vi "Constructor by Info Cluster Text.vi"(8 "error in (no error)":errorcluster, 9 "Text Field Info":T1, 10 "Database (use member data)":refnum<class "Database.lvclass">, 11 "Field in":refnum<class "Field.lvclass">) -> (0 "error out":errorcluster, 3 "Field out":refnum<class "Field.lvclass">)   [LabVIEW 2020, in "Old Field.lvlib" / "Field.lvclass"]
uses:
  Field.lvclass
  Database Libraries/Database/Database Class/Database.lvclass
  Text Field Info.ctl
  Basic Fields/Text field Class/Text field.lvclass
  C:/Users/User/Desktop/Raman Program/Database OOP/source/Database OOP/Field/Field Class/Field.lvclass
  Field.lvclass/Field.ctl
  Old Field.lvlib
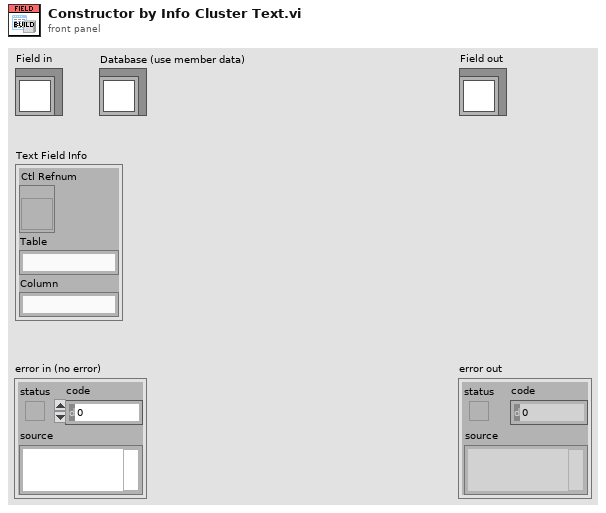
[diagram p1: front panel]
types:
  T1 = typedef "Old Field.lvlib/Text Field Info.ctl" = cluster{"Ctl Refnum":refnum<vi>, "Table":string, "Column":string}
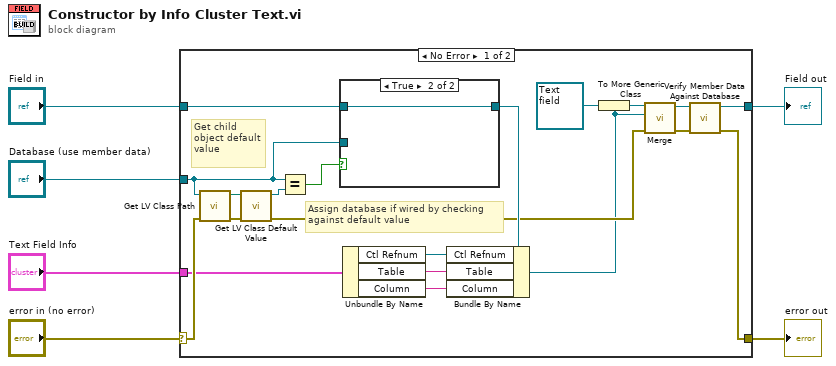
[diagram p0: block diagram]
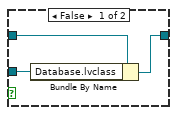
[diagram p2: hidden frame]
diagram:
  n1 = case shown="No Error" "error in (no error)" {
    selector: "error in (no error)" -> [w20 w32]
    tunnel: [w8 w32] -> w5
    tunnel: [w7 w31] -> w3
    tunnel: "Field in" -> [w21 w31]
    tunnel: "Database (use member data)" -> [w22 _]
    tunnel: "Text Field Info" -> [w17 _]
    frame No Error {
      # "Get child object default value"
      # "Assign database if wired by checking\nagainst default value"
      n2 = call <vilib>:"Get LV Class Path.vi"("error in (no error)"=w20, "object"=w22) -> ("error out"=w25:errorcluster, "class path"=w26:path)  [unwired: 8 in]
      n3 = call <vilib>:"Get LV Class Default Value.vi"("error in (no error)"=w25, "class path"=w26) -> ("error out"=w18:errorcluster, "object"=w24:refnum<class>)  [unwired: 8 in]
      n4 = Equal?(x=w22, y=w24) -> (x = y?=w23:bool)
      n5 = case shown="True" w23 {
        tunnel: w22 -> [w28 _]
        tunnel: w21 -> [w29 w30]
        tunnel: [w27 w30] -> w19
        frame False {
          n6 = Bundle By Name(cluster=w29, "Database.lvclass"=w28) -> (w27:refnum<class "Field.lvclass">)
        }
        frame True {
        }
      }
      n7 = Unbundle By Name(w17) -> ("Ctl Refnum"=w16:refnum<vi>, "Table"=w15:string, "Column"=w14:string)
      n8 = Bundle By Name(cluster=w19, "Ctl Refnum"=w16, "Table"=w15, "Column"=w14) -> (w12:refnum<class "Field.lvclass">)
      n9 = To More Generic Class(target class=w12, reference=refnum<class "Text field.lvclass"> refnum ("Text field.lvclass")) -> (generic class reference=w13:refnum<class "Field.lvclass">)
      n10 = call-dynamic "Merge.vi"("error in (no error)"=w18, "Field To Merge"=w12, "Field In"=w13) -> ("error out"=w9:errorcluster, "Merged Field out"=w10:refnum<class "Field.lvclass">)  [unwired: 7 in]
      n11 = call-dynamic "Verify Member Data Against Database.vi"("error in (no error)"=w9, "Field in"=w10) -> ("error out"=w8:errorcluster, "Field out"=w7:refnum<class "Field.lvclass">)  [unwired: 8 in]
    }
    frame Error {
    }
  }
  "error out" <- w5
  "Field out" <- w3
